vi "WFGenerate04FM.vi"(7 "Repetitions":T1={"Delay (s)"=0.0, "Interval (s)"=0.0, "Repeat"=1} {"Interval (s)" min=0.0; "Delay (s)" min=0.0}, 8 "error in (no error)":errorcluster, 9 "Waveform Properties":T3={"Fs (Hz)"=20000.0, "Amplitude (V)"=5.0, "Ramp (s)"=0.005, "Duration (s)"=0.25} {"Ramp (s)" min=0.0; "Fs (Hz)" min=0.0}, 10 "Waveform Parameters":T2={"Param 0: Start Hz"=2000.0, "Param 1: End Hz"=4000.0, "Param 2: Inactive"=0.0, "Param 3: Inactive"=0.0}) -> (0 "error out":errorcluster, 3 "Waveform Out":waveform(dbl))   [LabVIEW 2013]
panel:
  out "Waveform Graph":waveform(dbl)(graph)
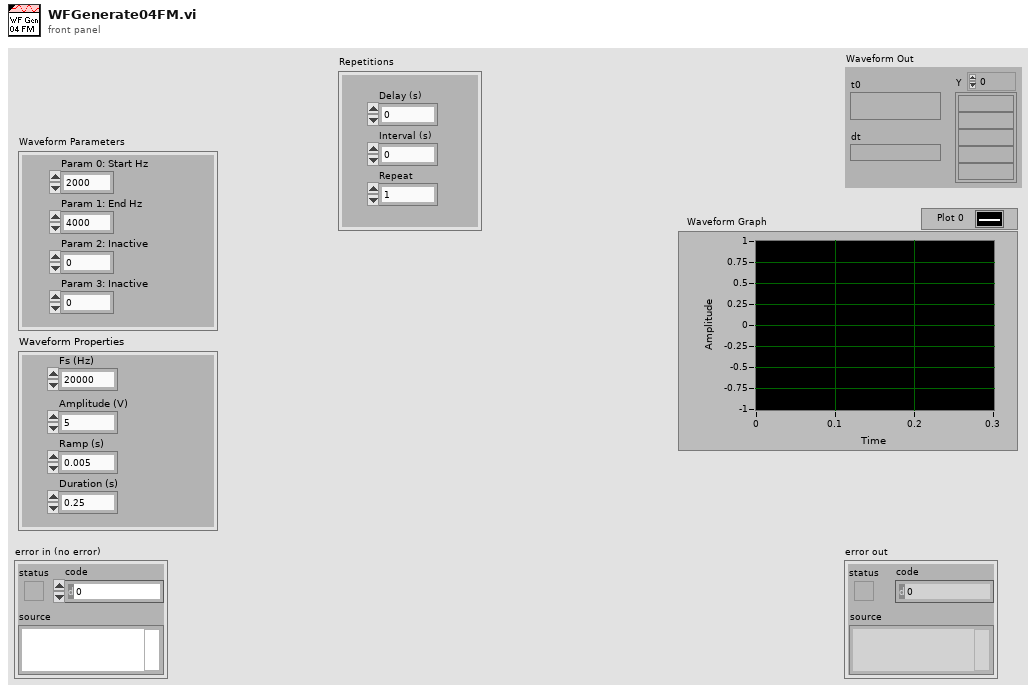
[diagram p1: front panel]
types:
  T1 = cluster{"Delay (s)":dbl, "Interval (s)":dbl, "Repeat":i32}
  T2 = cluster{"Param 0: Start Hz":dbl, "Param 1: End Hz":dbl, "Param 2: Inactive":dbl, "Param 3: Inactive":dbl}
  T3 = cluster{"Fs (Hz)":dbl, "Amplitude (V)":dbl, "Ramp (s)":dbl, "Duration (s)":dbl}
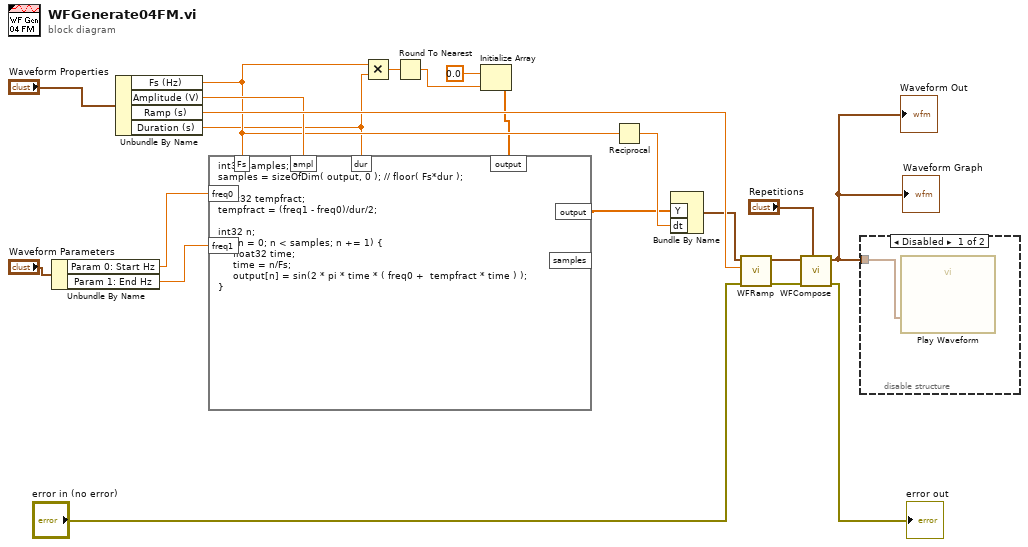
[diagram p0: block diagram]
diagram:
  n1 = Unbundle By Name("Waveform Parameters") -> ("Param 0: Start Hz"=w7:dbl, "Param 1: End Hz"=w6:dbl)
  n2 = Unbundle By Name("Waveform Properties") -> ("Fs (Hz)"=w15:dbl, "Amplitude (V)"=w20:dbl, "Ramp (s)"=w21:dbl, "Duration (s)"=w10:dbl)
  n3 = Multiply(x=w15, y=w10) -> (x*y=w14:dbl)
  n4 = Round To Nearest(number=w14) -> (nearest integer value=w13:dbl)
  n5 = Initialize Array(0.0 ("element"), w13) -> (w12:dbl[])
  n6 = formula code="int32 samples;\nsamples = sizeOfDim( output, 0 ); // floor( Fs*dur );\n\nfloat32 tempfract;\ntempfract = (freq1 - freq0)/dur/2;\n\nint32 n;\nfor( n = 0; n < samples; n += 1) {\n     float32 time;\n     time = n/Fs;\n     output[n] = sin(2 * pi * time * ( freq0 +  tempfract * time ) );\n}"("dur"=w10, "freq0"=w7, "freq1"=w6, "ampl"=w20, "Fs"=w15, "output"=w12) -> ("output"=w17:dbl[])  [unwired: 1 out]
  n7 = Reciprocal(x=w15) -> (1/x=w19:dbl)
  n8 = Bundle By Name("Y"=w17, "dt"=w19) -> (w18:waveform(dbl))  [unwired: 1 in]
  n9 = call "WFRamp.vi"("error in (no error)"="error in (no error)", "Ramp Length (s)"=w21, "Waveform In"=w18) -> ("error out"=w4:errorcluster, "Waveform Out"=w5:waveform(dbl))  [unwired: 7 in]
  n10 = call "WFCompose.vi"("Repetitions"="Repetitions", "error in (no error)"=w4, "Waveform In"=w5) -> ("error out"=→"error out":errorcluster, "Analog Waveform Out"=w1:waveform(dbl))  [unwired: 7 in]
  "Waveform Out" <- w1
  "Waveform Graph" <- w1
  n11 = disable-structure shown="Disabled" {
    disable-tunnel: w1 -> [w22 _]
    frame Disabled {
      n12 = call "Play Waveform"("Data"=w22) -> ()  [unwired: 18 in, 1 out]
    }
    frame Enabled {
    }
  }
